vi "DAQmxCreateVC(SubVI).vi"(6 "line grouping":i32(ring)=1 items=["one channel for each line", "one channel for all lines"], 7 "index":i32, 8 "error in (no error)":errorcluster, 9 "Device Name":string, 10 "Physical Channels":string[](array[string]), 11 "Refnum in":refnum<k21>) -> (0 "error out":errorcluster, 2 "line grouping":i32, 3 "Refnum out":refnum<k21>)   [LabVIEW 2015]
uses:
  <vilib>/DAQmx/create/channels.llb/DAQmx Create Channel (DO-Digital Output).vi
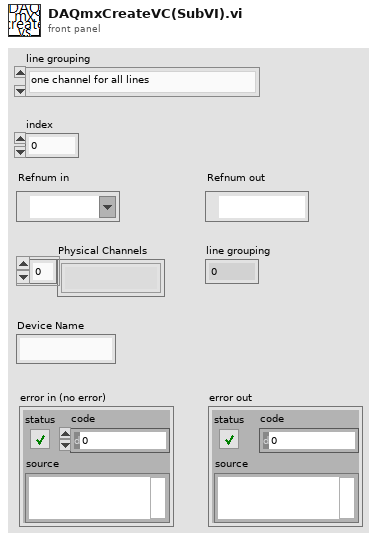
[diagram p1: front panel]
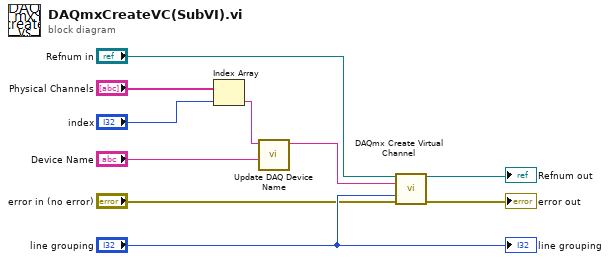
[diagram p0: block diagram]
diagram:
  n1 = Index Array(array="Physical Channels", index="index") -> (element=w8:string)
  n2 = call "Update DAQ Device Name.vi"("Device Name"="Device Name", "Lines in (String)"=w8) -> ("Lines out (DAQmx Physical Channels)"=w9:tag)  [unwired: 9 in]
  n3 = call-poly <vilib>:"DAQmx Create Virtual Channel.vi"("task in"="Refnum in", "lines"=w9, "line grouping"="line grouping", "error in"="error in (no error)") -> ("task out"=→"Refnum out":refnum<k21>, "error out"=→"error out":errorcluster)  [unwired: 10 in]
  "line grouping" <- "line grouping"
